vi "Initialize Osciloscope.vi"(8 "error in (no error)":errorcluster, 10 "Initialize--cluster":T1={"TEKTRONIX-INITIALIZE"={"ID Query? (T: Yes)"=TRUE, "Reset? (T: Yes)"=TRUE, "Serial-Configuration"={"Baud Rate"=9600, "Parity"=0, "Stop Bits"=10, "Flow Control"=2}}, "EDU-X-1200A- INITIALIZE"={"Reset (True)"=TRUE, "ID Query (True)"=TRUE}} {"TEKTRONIX-INITIALIZE"."Serial-Configuration"."Flow Control" items=["None", "XON/XOFF", "RTS/CTS", "XON/XOFF & RTS/CTS", "DTR/DSR", "XON/XOFF & DTR/DSR"]; "TEKTRONIX-INITIALIZE"."Serial-Configuration"."Stop Bits" items=["1.0"=10, "1.5"=15, "2.0"=20]; "TEKTRONIX-INITIALIZE"."Serial-Configuration"."Parity" items=["None", "Odd", "Even", "Mark", "Space"]; "TEKTRONIX-INITIALIZE"."Serial-Configuration"."Baud Rate" items=["300"=300, "600"=600, "1200"=1200, "2400"=2400, "4800"=4800, "9600"=9600, "19200"=19200]}, 11 "EDU-X 1002A in":refnum<class "EDU-X 1002A.lvclass">) -> (0 "error out":errorcluster, 3 "EDU-X 1002A out":refnum<class "EDU-X 1002A.lvclass">)   [LabVIEW 2020, in "EDU-X 1002A.lvclass"]
uses:
  EDU-X 1002A.lvclass
  TypeDefs/InitializeOsciloscope--cluster.ctl
  EDU-X 1002A.lvclass/EDU-X 1002A.ctl
  <instrlib>/Agilent 2000 3000 X-Series/Agilent 2000 3000 X-Series.lvlib
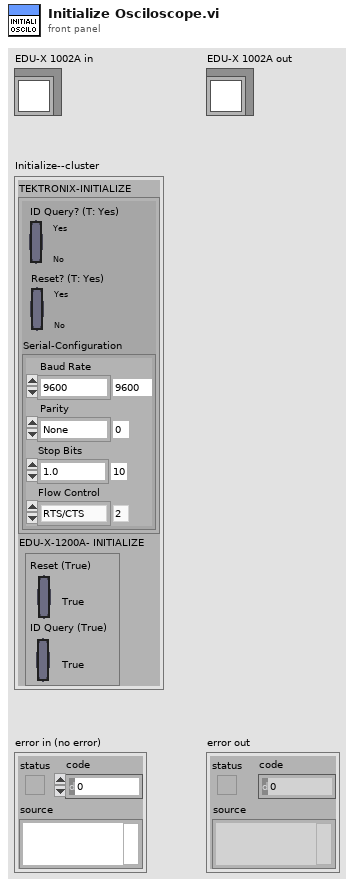
[diagram p1: front panel]
types:
  T1 = typedef "InitializeOsciloscope--cluster.ctl" = cluster{"TEKTRONIX-INITIALIZE":cluster{"ID Query? (T: Yes)":bool, "Reset? (T: Yes)":bool, "Serial-Configuration":cluster{"Baud Rate":u32, "Parity":u16, "Stop Bits":u16, "Flow Control":u16}}, "EDU-X-1200A- INITIALIZE":cluster{"Reset (True)":bool, "ID Query (True)":bool}}
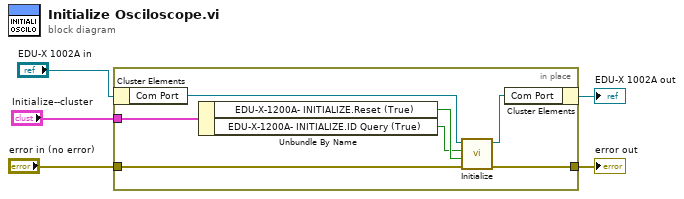
[diagram p0: block diagram]
diagram:
  n1 = in-place {
    in-place-border: [w10] -> w3
    in-place-border: "error in (no error)" -> [w9]
    in-place-border: "Initialize--cluster" -> [w8]
    n2 = in-place-cluster #1("EDU-X 1002A in") -> ("Com Port"=w12:refnum<visa-resource-name>)
    n3 = Unbundle By Name(w8) -> ("EDU-X-1200A- INITIALIZE.Reset (True)"=w7:bool, "EDU-X-1200A- INITIALIZE.ID Query (True)"=w6:bool)
    n4 = call <instrlib>:"Initialize.vi"("error in (no error)"=w9, "Reset (True)"=w7, "ID Query (True)"=w6, "VISA resource name"=w12) -> ("error out"=w10:errorcluster, "VISA resource name out"=w11:refnum<visa-resource-name>)  [unwired: 6 in]
    n5 = in-place-cluster #1("Com Port"=w11) -> (→"EDU-X 1002A out":refnum<class "EDU-X 1002A.lvclass">)
  }
  "error out" <- w3
